vi "dfd_Convert String to Filter.vi"(7 "load type":T7 items=["From Coef", "From ZPK"], 8 "error in (no error)":errorcluster, 10 "xml string":string, 11 "filter in":T1={"mSRate_Fs"=1.0, "mSRate_Version"="1.0", "mSRate_Comments"="", "mSRate_OrgCoef"={"type"=enum."Undefined", "gain"=1.0, "coef a (k)"=[], "coef b (v)"=[]}, "mSRate_CurCoef"={"type"=enum."Undefined", "gain"=1.0, "coef a (k)"=[], "coef b (v)"=[]}, "mSRate_Quantized?"=FALSE, "mSRate_QCoef"={"type"=enum."Undefined", "gain"=1.0, "coef a (k)"=[], "coef b (v)"=[]}, "mSRate_QSettings"=[], "mSRate_Order"=0, "mSRate_Scaling"={"mSRate_ScaleByPowerOf2?"=FALSE, "mSRate_ScaleType"=enum."No Norm"}} {"mSRate_QSettings"."source" items=["Coef a/k"=0, "Coef b/v"=7, "Input"=1, "Output"=2, "Multiplicand"=3, "Product"=4, "Sum"=5, "Delay"=6, "Gain"=8]}) -> (0 "error out":errorcluster, 3 "filter out":T1={"mSRate_Fs"=1.0, "mSRate_Version"="1.0", "mSRate_Comments"="", "mSRate_OrgCoef"={"type"=enum."Undefined", "gain"=1.0, "coef a (k)"=[], "coef b (v)"=[]}, "mSRate_CurCoef"={"type"=enum."Undefined", "gain"=1.0, "coef a (k)"=[], "coef b (v)"=[]}, "mSRate_Quantized?"=FALSE, "mSRate_QCoef"={"type"=enum."Undefined", "gain"=1.0, "coef a (k)"=[], "coef b (v)"=[]}, "mSRate_QSettings"=[], "mSRate_Order"=0, "mSRate_Scaling"={"mSRate_ScaleByPowerOf2?"=FALSE, "mSRate_ScaleType"=enum."No Norm"}} {"mSRate_QSettings"."source" items=["Coef a/k"=0, "Coef b/v"=7, "Input"=1, "Output"=2, "Multiplicand"=3, "Product"=4, "Sum"=5, "Delay"=6, "Gain"=8]})   [LabVIEW 2017, in "NI_DigFilter_Process.lvlib"]
uses:
  <vilib>/addons/Digital Filter Design/NI_DigFilter_Process.lvlib
  <vilib>/addons/Digital Filter Design/_Objects.llb/DFD Filter Obj.ctl
  <vilib>/addons/Digital Filter Design/_Objects.llb/DFD Filter Coef.ctl
  <vilib>/addons/Digital Filter Design/_Objects.llb/DFD Filter Structure Type Selector.ctl
  <vilib>/addons/Digital Filter Design/_Objects.llb/dfd_Internal Quantization Settings.ctl
  <vilib>/addons/Digital Filter Design/_Objects.llb/dfd_Internal Quantization Srcs.ctl
  <vilib>/addons/Digital Filter Design/_Objects.llb/DFD Coef Norm Type.ctl
  <vilib>/addons/Digital Filter Design/_TextIOUtils.llb/dfd_Load Type.ctl
  <vilib>/addons/Digital Filter Design/NI_DigFilterLicensed.lvlib
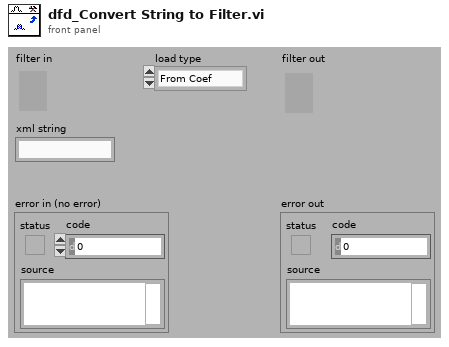
[diagram p1: front panel]
types:
  T1 = typedef "NI_DigFilterLicensed.lvlib/DFD Filter Obj.ctl" = cluster{"mSRate_Fs":dbl, "mSRate_Version":string, "mSRate_Comments":string, "mSRate_OrgCoef":T2, "mSRate_CurCoef":T2, "mSRate_Quantized?":bool, "mSRate_QCoef":T2, "mSRate_QSettings":T4[], "mSRate_Order":i32, "mSRate_Scaling":cluster{"mSRate_ScaleByPowerOf2?":bool, "mSRate_ScaleType":T6}}
  T2 = typedef "NI_DigFilterLicensed.lvlib/DFD Filter Coef.ctl" = cluster{"type":T3, "gain":dbl, "coef a (k)":dbl[], "coef b (v)":dbl[]}
  T3 = typedef "NI_DigFilterLicensed.lvlib/DFD Filter Structure Type Selector.ctl" = enum16{"Undefined", "FIR Direct Form", "FIR Direct Form Transposed", "FIR Symmetric", "FIR Antisymmetric", "IIR Direct Form I", "IIR Direct Form I Transposed", "IIR Direct Form II", "IIR Direct Form II Transposed", "IIR Cascaded Second Order Sections Form I", "IIR Cascaded Second Order Sections Form I Transposed", "IIR Cascaded Second Order Sections Form II", "IIR Cascaded Second Order Sections Form II Transposed", "Lattice Allpass (basic sections)", "Lattice Allpass (one multiplier sections)", "Lattice Allpass (normalized sections)", "Lattice AR (basic sections)", "Lattice AR (one multiplier sections)", "Lattice AR (normalized sections)", "Lattice MA (minimum phase)", "Lattice MA (maximum phase)", "Lattice ARMA (basic sections)", "Lattice ARMA (one multiplier sections)", "Lattice ARMA (normalized sections)"}
  T4 = typedef "NI_DigFilterLicensed.lvlib/dfd_Internal Quantization Settings.ctl" = cluster{"source":T5, "wl":i16, "iwl":i16, "overflow mode":enum16{"Saturation", "Wrap"}, "rounding mode":enum16{"Nearest", "Truncation"}, "signed?":bool}
  T5 = typedef "NI_DigFilterLicensed.lvlib/dfd_Internal Quantization Srcs.ctl" = u16
  T6 = typedef "NI_DigFilterLicensed.lvlib/DFD Coef Norm Type.ctl" = enum16{"No Norm", "Time Domain 1-Norm", "Time Domain 2-Norm", "Time Domain Inf-Norm"}
  T7 = typedef "dfd_Load Type.ctl" = u16
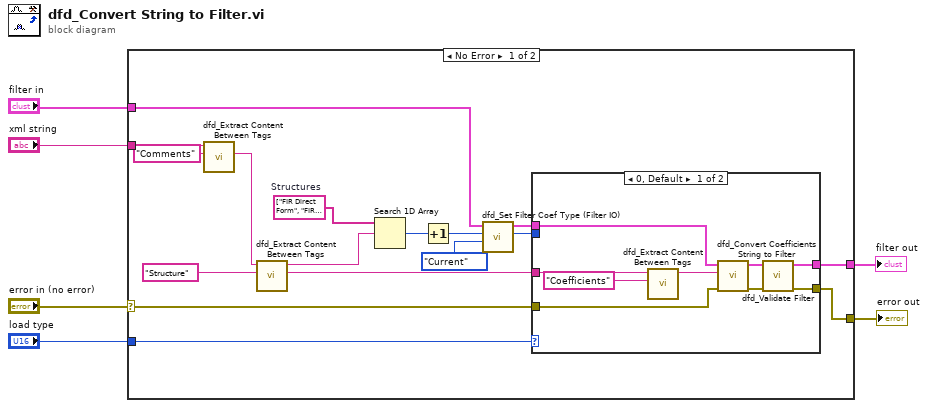
[diagram p0: block diagram]
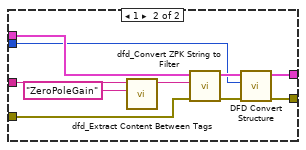
[diagram p2: hidden frame]
diagram:
  n1 = case shown="No Error" "error in (no error)" {
    selector: "error in (no error)" -> [w16 w43]
    tunnel: "xml string" -> [w22 _]
    tunnel: "filter in" -> [w12 w42]
    tunnel: [w8 w42] -> w5
    tunnel: [w9 w43] -> w4
    tunnel: "load type" -> [w15 _]
    frame No Error {
      w7 = string[] ["FIR Direct Form", "FIR Direct Form Transposed", "FIR Symmetric", "FIR Antisymmetric", "IIR Direct Form I", "IIR Direct Form I Transposed", "IIR Direct Form II", "IIR Direct Form II Transposed", "IIR Cascaded Second-Order Sections Form I", "IIR Cascaded Second-Order Sections Form I Transposed", "IIR Cascaded Second-Order Sections Form II", "IIR Cascaded Second-Order Sections Form II Transposed", "Lattice Allpass (basic sections)", "Lattice Allpass (one multiplier sections)", "Lattice Allpass (normalized sections)", "Lattice AR (basic sections)", "Lattice AR (one multiplier sections)", "Lattice AR (normalized sections)", "Lattice MA (minimum phase)", "Lattice MA (maximum phase)", "Lattice ARMA (basic sections)", "Lattice ARMA (one multiplier sections)", "Lattice ARMA (normalized sections)"]  # Structures
      n2 = call <vilib>:"dfd_Extract Content Between Tags.vi"("element"="Comments", "xml string with tag"=w22) -> ("remaining string"=w19:string)  [unwired: 9 out]
      n3 = call <vilib>:"dfd_Extract Content Between Tags.vi"("element"="Structure", "xml string with tag"=w19) -> ("remaining string"=w18:string, "content"=w17:string)  [unwired: 8 out]
      n4 = Search 1D Array(1D array=w7, element=w17) -> (index of element=w14:i32)  [unwired: 1 out]
      n5 = Increment(x=w14) -> (x+1=w10:i32)
      n6 = call <vilib>:"dfd_Set Filter Coef Type (Filter IO).vi"("coef source"=enum16{"Original", "Current", "Quantized"}."Current", "type"=w10, "filter in"=w12) -> ("filter out"=w13:T1)  [unwired: 1 in, 7 out]
      n7 = case shown="0, Default" w15 {
        tunnel: w18 -> [w31 w41]
        tunnel: w16 -> [w28 w39]
        tunnel: [w24 w37] -> w8
        tunnel: [w23 w34] -> w9
        tunnel: w13 -> [w27 w33]
        tunnel: w10 -> [_ w32]
        frame 0, Default {
          n8 = call <vilib>:"dfd_Extract Content Between Tags.vi"("element"="Coefficients", "xml string with tag"=w31) -> ("content"=w29:string)  [unwired: 9 out]
          n9 = call <vilib>:"dfd_Convert Coefficients String to Filter.vi"("error in (no error)"=w28, "xml string in"=w29, "filter"=w27) -> ("error out"=w25:errorcluster, "filter out"=w26:T1)  [unwired: 7 out]
          n10 = call <vilib>:"dfd_Validate Filter.vi"("error in (no error)"=w25, "filter in"=w26) -> ("error out"=w23:errorcluster, "filter out"=w24:T1)  [unwired: 1 in, 7 out]
        }
        frame 1 {
          n11 = call <vilib>:"dfd_Extract Content Between Tags.vi"("element"="ZeroPoleGain", "xml string with tag"=w41) -> ("content"=w38:string)  [unwired: 9 out]
          n12 = call <vilib>:"dfd_Convert ZPK String to Filter.vi"("error in (no error)"=w39, "xml string in"=w38, "filter"=w33) -> ("error out"=w35:errorcluster, "filter out"=w36:T1)  [unwired: 7 out]
          n13 = call <vilib>:"DFD Convert Structure.vi"("error in (no error)"=w35, "target structure"=w32, "filter in"=w36) -> ("error out"=w34:errorcluster, "filter out"=w37:T1)  [unwired: 7 out]
        }
      }
    }
    frame Error {
    }
  }
  "filter out" <- w5
  "error out" <- w4
